vi "Message.vi"(8 "error in":errorcluster, 11 "Node Ptr":T1 format="%.0x") -> (0 "error out":errorcluster)   [LabVIEW 2020, in "AIM MIL-STD-1553 System Explorer.lvlib" / "Implementation.lvlib"]
uses:
  Implementation.lvlib
  <vilib>/NI VeriStand/Custom Device API/Custom Device Item Ref.ctl
  <vilib>/NI VeriStand/Custom Device API/Custom Device API.lvlib
panel:
  in  "SHDocVw.IWebBrowser":refnum<k7>(container)
  in  "General Header":cluster{"Section Name":string}={"Section Name"="AIM MIL-STD 1553 - Message"}
  in  "Description":string
  out "Name":string
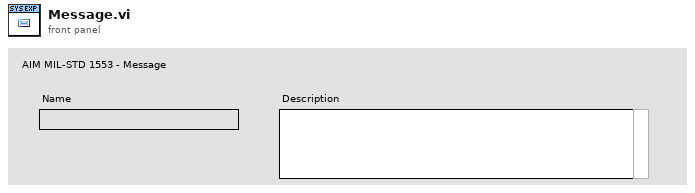
[diagram p1: front panel]
types:
  T1 = typedef "Custom Device API.lvlib/Custom Device Item Ref.ctl" = u64
  T2 = typedef "Custom Device API.lvlib/Custom Device Item Info.ctl" = cluster{"Name":string, "Is Channel":bool, "GUID":string, "Is Waveform":bool}
  T3 = typedef "Custom Device API.lvlib/Custom Device Commands.ctl" = enum16{"Default", "Item renamed", "Shutdown", "Dynamic button pressed"}
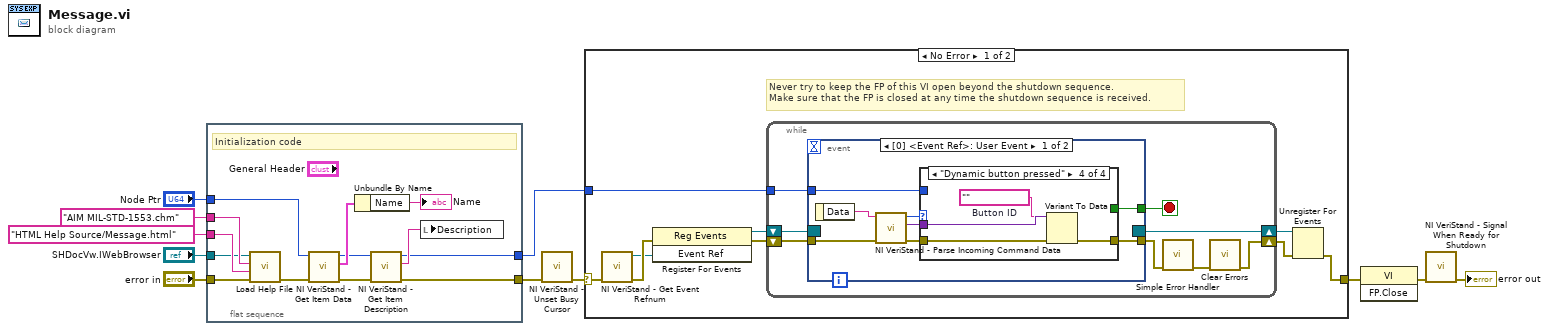
[diagram p0: block diagram]
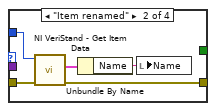
[diagram p3: hidden frame]
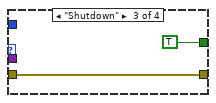
[diagram p4: hidden frame]
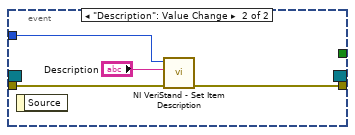
[diagram p5: hidden frame]
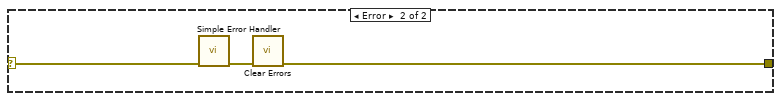
[diagram p6: hidden frame]
diagram:
  n1 = flat-sequence "Initialization code" {
    tunnel: "error in" -> [w22]
    tunnel: "Node Ptr" -> [w17]
    tunnel: [w13] -> w7
    tunnel: [w12] -> w4
    tunnel: "SHDocVw.IWebBrowser" -> [w19]
    tunnel: "HTML Help Source/Message.html" ("CD_CHM_Section") -> [w21]
    tunnel: "AIM MIL-STD-1553.chm" ("CD_CHM_FileName") -> [w20]
    frame #0 {
      # "Initialization code"
      n2 = call "Load Help File.vi"("error in (no error)"=w22, "HTML File to Load"=w21, "Main CHM File"=w20, "Browser"=w19) -> ("error out"=w16:errorcluster)  [unwired: 7 in]
      n3 = call <vilib>:"NI VeriStand - Get Item Data.vi"("error in (no error)"=w16, "Item Ref in"=w17) -> ("error out"=w14:errorcluster, "Item Info"=w24:T2, "Item Ref out"=w15:T1)  [unwired: 7 out]
      n4 = Unbundle By Name(w24) -> ("Name"=→"Name":string)
      n5 = call <vilib>:"NI VeriStand - Get Item Description.vi"("error in (no error)"=w14, "Item Ref in"=w15) -> ("error out"=w13:errorcluster, "Description"=w23:string, "Item Ref out"=w12:T1)  [unwired: 7 out]
      n6 = local write "Description"(w23) -> ()
    }
  }
  n7 = call <vilib>:"NI VeriStand - Unset Busy Cursor.vi"("error in (no error)"=w7) -> ("error out"=w6:errorcluster)  [unwired: 10 out]
  n8 = case shown="No Error" w6 {
    selector: w6 -> [w25 w68]
    tunnel: [w30 w66] -> w11
    tunnel: w4 -> [w26 _]
    frame No Error {
      # "Never try to keep the FP of this VI open beyond the shutdown sequence.\nMake sure that the FP is closed at any time the shutdown sequence is received."
      n9 = call <vilib>:"NI VeriStand - Get Event Refnum.vi"("error in (no error)"=w25) -> ("error out"=w33:errorcluster, "Event Ref"=w29:refnum<user-event>)  [unwired: 9 out]
      n10 = register-events(error in=w33, w29) -> (reference out=w27:refnum<event-registration>, error out=w28:errorcluster)  [unwired: 1 in]
      n11 = while {
        tunnel: w26 -> [w37]
        shift-right: [w34] -> w31
        shift-left: w28 -> [w40]
        shift-right: [w41] -> w32
        shift-left: w27 -> [w39]
        stop <- w38 stop-if-true
        n12 = event shown="[0] <Event Ref>: User Event" {
          selector: w39 -> [_ _]
          dyn-events: [_ _] -> w41
          timeout: _ -> [_ _]
          tunnel: w40 -> [w49 w64]
          tunnel: [w46 _] -> w38
          tunnel: [w45 w63] -> w36
          tunnel: w37 -> [w44 w65]
          event User Event {
            n13 = event-data() -> ("Data"=w42:string)  [unwired: 1 out]
            n14 = call <vilib>:"NI VeriStand - Parse Incoming Command Data.vi"("error in (no error)"=w49, "Incoming data"=w42) -> ("error out"=w48:errorcluster, "Outgoing data"=w43:variant, "Action"=w47:T3)  [unwired: 7 out]
            n15 = case shown="\"Dynamic button pressed\"" w47 {
              tunnel: w48 -> [w50 w55 w56 w61]
              tunnel: [_ _ TRUE _] -> w46
              tunnel: [w50 w52 w56 w58] -> w45
              tunnel: w44 -> [_ w54 _ _]
              tunnel: w43 -> [_ _ _ w60]
              frame Default {
              }
              frame "Item renamed" {
                n16 = call <vilib>:"NI VeriStand - Get Item Data.vi"("error in (no error)"=w55, "Item Ref in"=w54) -> ("error out"=w52:errorcluster, "Item Info"=w53:T2)  [unwired: 8 out]
                n17 = Unbundle By Name(w53) -> ("Name"=w51:string)
                n18 = local write "Name"(w51) -> ()
              }
              frame "Shutdown" {
              }
              frame "Dynamic button pressed" {
                w59 = ""  # Button ID
                n19 = Variant To Data(error in=w61, type=w59, Variant=w60) -> (error out=w58:errorcluster)  [unwired: 1 out]
              }
            }
          }
          event "Description": Value Change {
            n20 = event-data() -> ()  [unwired: 2 out]
            n21 = call <vilib>:"NI VeriStand - Set Item Description.vi"("error in (no error)"=w64, "Description"="Description", "Item Ref in"=w65) -> ("error out"=w63:errorcluster)  [unwired: 8 out]
          }
        }
        n22 = call <vilib>:"Simple Error Handler.vi"("error in (no error)"=w36) -> ("error out"=w35:errorcluster)  [unwired: 1 in, 7 out]
        n23 = call <vilib>:"Clear Errors.vi"("error in (no error)"=w35) -> ("error out"=w34:errorcluster)  [unwired: 1 in, 5 out]
      }
      n24 = Unregister For Events(event registration refnum=w32, error in=w31) -> (error out=w30:errorcluster)
    }
    frame Error {
      n25 = call <vilib>:"Simple Error Handler.vi"("error in (no error)"=w68) -> ("error out"=w67:errorcluster)  [unwired: 1 in, 7 out]
      n26 = call <vilib>:"Clear Errors.vi"("error in (no error)"=w67) -> ("error out"=w66:errorcluster)  [unwired: 1 in, 5 out]
    }
  }
  n27 = invoke class="VI" method="FP.Close"(error in=w11) -> (error out=w10:errorcluster)  [unwired: 2 in, 2 out]
  n28 = call <vilib>:"NI VeriStand - Signal When Ready for Shutdown.vi"("error in (no error)"=w10) -> ("error out"=→"error out":errorcluster)  [unwired: 10 out]
